vi "4.7.vi"() -> (0 "输入1-1000":dbl format="%#g", 1 "数值":i32, 2 "数值 2":i32)   [LabVIEW 2017]
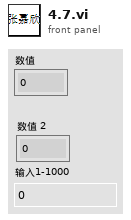
[diagram p1: front panel]
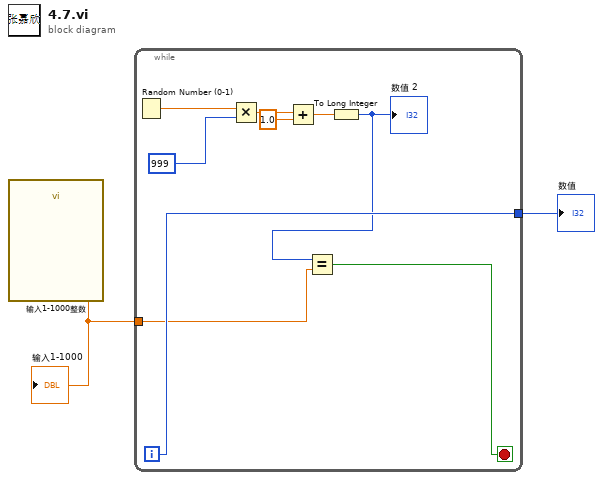
[diagram p0: block diagram]
diagram:
  n1 = call "输入1-1000整数"() -> ("输入1-1000"=w1:dbl)  [unwired: 17 in, 2 out]
  "输入1-1000" <- w1
  n2 = while {
    tunnel: [w9] -> w2
    tunnel: w1 -> [w7]
    i -> [w9]
    stop <- w8 stop-if-true
    n3 = Random Number (0-1)() -> (number: 0 to 1=w11:dbl)
    n4 = Multiply(x=w11, y=999) -> (x*y=w6:dbl)
    n5 = Add(x=w6, y=1.0) -> (x+y=w4:dbl)
    n6 = To Long Integer(number=w4) -> (32bit integer=w3:i32)
    "数值 2" <- w3
    n7 = Equal?(x=w3, y=w7) -> (x = y?=w8:bool)
  }
  "数值" <- w2
